vi "Get Registry Configuration.vi"(8 "error in (no error)":errorcluster, 11 "Registry in":refnum<data-value>) -> (0 "error out":errorcluster, 2 "Registry Configuration":T1, 3 "Registry":refnum<data-value>)   [LabVIEW 2014, in "UniqueName.lvlib" / "NameRegistry.lvclass"]
uses:
  NameRegistry.lvclass
  RegistryConfiguration.ctl
  Delimiter/Delimiter.lvclass
  RandomStringGenerator/RandomStringGenerator.lvclass
  UniquenessCriteria/UniquenessCriteria.lvclass
  StringIncrement/StringIncrement.lvclass
  NameRegistry.lvclass/NameRegistry.ctl
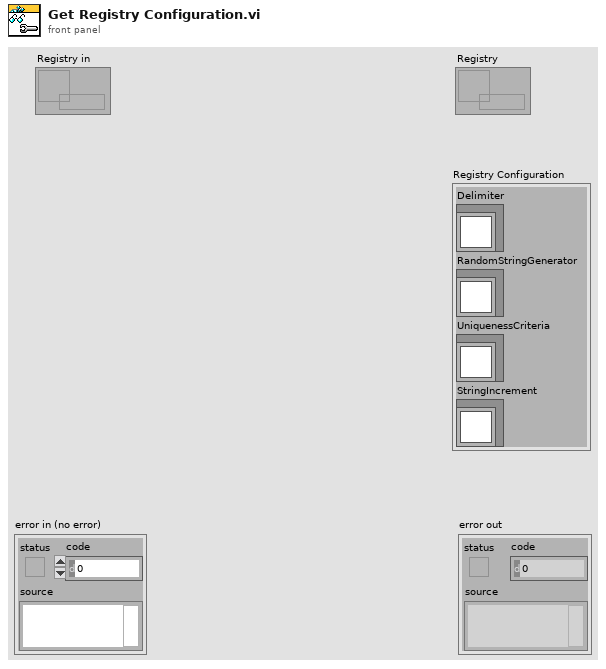
[diagram p1: front panel]
types:
  T1 = typedef "UniqueName.lvlib/NameRegistry.lvclass/RegistryConfiguration.ctl" = cluster{"Delimiter":refnum<class "Delimiter.lvclass">, "RandomStringGenerator":refnum<class "RandomStringGenerator.lvclass">, "UniquenessCriteria":refnum<class "UniquenessCriteria.lvclass">, "StringIncrement":refnum<class "StringIncrement.lvclass">}
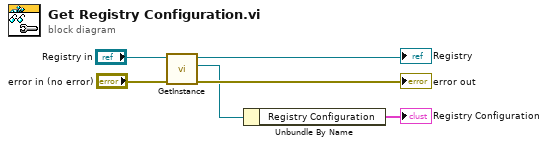
[diagram p0: block diagram]
diagram:
  n1 = call "GetInstance.vi"("error in (no error)"="error in (no error)", "Registry in"="Registry in") -> ("error out"=→"error out":errorcluster, "Instance"=w1:refnum<class "NameRegistry.lvclass">, "Registry out"=→"Registry":refnum<data-value>)  [unwired: 7 in]
  n2 = Unbundle By Name(w1) -> ("Registry Configuration"=→"Registry Configuration":T1)
